vi "ParsePOXData.vi"(10 "POX Data in":string) -> (1 "O2":dbl, 2 "Hear Beat":dbl, 5 "Valid?":bool)   [LabVIEW 2019]
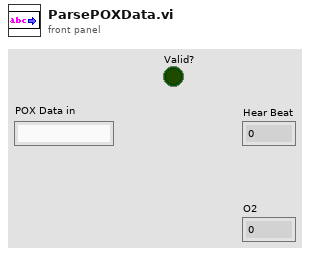
[diagram p1: front panel]
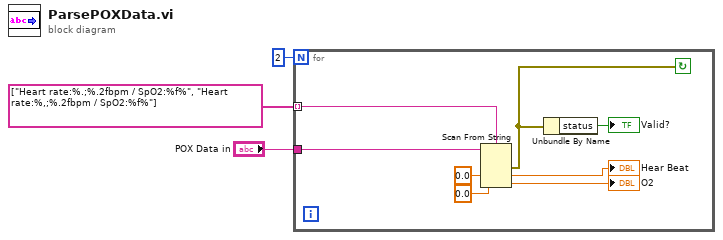
[diagram p0: block diagram]
diagram:
  n1 = for {
    N: 2 -> [_]
    tunnel: "POX Data in" -> [w11]
    tunnel: string[] ["Heart rate:%.;%.2fbpm / SpO2:%f%", "Heart rate:%,;%.2fbpm / SpO2:%f%"] ("format string") -> [w4] mode=indexing
    stop <- w5 continue-if-true
    n2 = Scan From String(format string=w4, input string=w11, default 1=0.0 ("default value 1"), default 2=0.0 ("default value 2")) -> (error out=w5:errorcluster, output 1=→"Hear Beat":dbl, output 2=→"O2":dbl)  [unwired: 2 in, 2 out]
    n3 = Unbundle By Name(w5) -> ("status"=→"Valid?":bool)
  }
